vi "Config Input Settings.vi"(0 "VISA resource name":refnum<visa-resource-name>, 1 "Scan Dwell Time (10)":dbl=10.0 min=1.0 max=200.0 step=1.0, 2 "Change Pause Time (3)":dbl=3.0 min=3.0 max=200.0 step=1.0, 5 "Channel (1)":i32=1 min=0 max=16 step=1, 7 "Channel On/Off (T: ON)":bool=TRUE, 9 "Curve Number (0)":dbl min=0.0 max=20.0 step=1.0, 11 "error in (no error)":errorcluster, 12 "Temperature Coefficient (0: Negative)":u16(ring) items=["Negative", "Positive"]) -> (4 "VISA resource name out":refnum<visa-resource-name>, 15 "error out":errorcluster)   [LabVIEW 2025, in "Lake Shore Cryotronics 370.lvlib"]
doc: "This VI configures the 370 input setup. The input parameters configured are channel off/on, scan dwell time, change pause time, curve number, and temperature coefficient."
uses:
  Lake Shore Cryotronics 370.lvlib
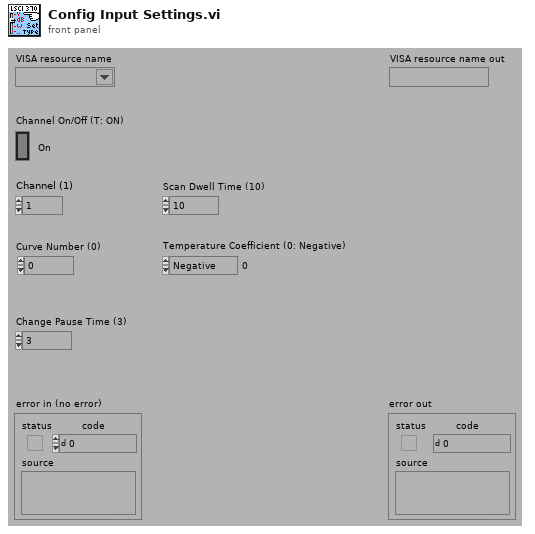
[diagram p1: front panel]
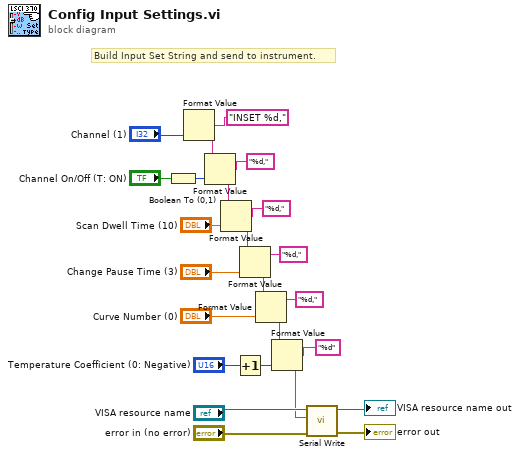
[diagram p0: block diagram]
diagram:
  # "Build Input Set String and send to instrument."
  n1 = Boolean To (0,1)(Boolean="Channel On/Off (T: ON)") -> (0, 1=w10:i16)
  n2 = Format Value(format string="INSET %d,", value (0)="Channel (1)") -> (output string=w12:string)  [unwired: 1 in]
  n3 = Format Value(string ("")=w12, format string="%d,", value (0)=w10) -> (output string=w9:string)
  n4 = Format Value(string ("")=w9, format string="%d,", value (0)="Scan Dwell Time (10)") -> (output string=w17:string)
  n5 = Increment(x="Temperature Coefficient (0: Negative)") -> (x+1=w1:u16)
  n6 = Format Value(string ("")=w17, format string="%d,", value (0)="Change Pause Time (3)") -> (output string=w6:string)
  n7 = Format Value(string ("")=w6, format string="%d,", value (0)="Curve Number (0)") -> (output string=w5:string)
  n8 = Format Value(string ("")=w5, format string="%d", value (0)=w1) -> (output string=w16:string)
  n9 = call "Serial Write.vi"("error in (no error)"="error in (no error)", "Write Buffer (\"\")"=w16, "VISA resource name"="VISA resource name") -> ("error out"=→"error out":errorcluster, "VISA resource name out"=→"VISA resource name out":refnum<visa-resource-name>)  [unwired: 6 in, 1 out]
